vi "Camera.vi"(11 "test mode":bool) -> (1 "Error":bool)   [LabVIEW 2020]
panel:
  out "standard output":string caption="Standardausgabe"
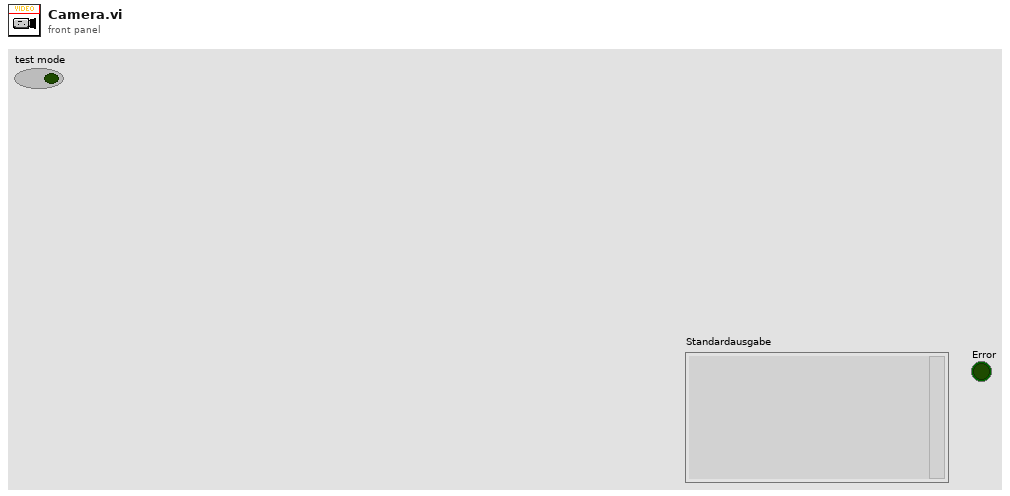
[diagram p1: front panel]
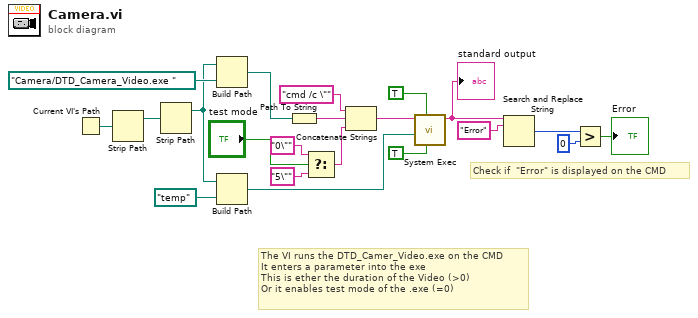
[diagram p0: block diagram]
diagram:
  # "Check if  \"Error\" is displayed on the CMD"
  # "The VI runs the DTD_Camer_Video.exe on the CMD\nIt enters a parameter into the exe\nThis is ether the duration of the Video (>0)\nOr it enables test mode of the .exe (=0)"
  n1 = Current VI's Path() -> (path=w10:path)
  n2 = Strip Path(path=w10) -> (stripped path=w9:path)  [unwired: 1 out]
  n3 = Strip Path(path=w9) -> (stripped path=w3:path)  [unwired: 1 out]
  n4 = Build Path(base path=w3, name or relative path=path "Camera/DTD_Camera_Video.exe ") -> (appended path=w18:path)
  n5 = Build Path(base path=w3, name or relative path=path "temp") -> (appended path=w1:path)
  n6 = Path To String(path=w18) -> (string=w17:string)
  n7 = Select(t="0\"" ("string"), s="test mode", f="5\"" ("string")) -> (s? t:f=w16:string)
  n8 = Concatenate Strings("cmd /c \"" ("string"), w17, w16) -> (w11:string)
  n9 = call <vilib>:"System Exec.vi"("run minimized? (F)"=TRUE, "wait until completion? (T)"=TRUE, "working directory"=w1, "command line"=w11) -> ("standard output"=w4:string)  [unwired: 4 in, 3 out]
  "standard output" <- w4
  n10 = Search and Replace String(input string=w4, search string="Error") -> (number of replacements=w7:i32)  [unwired: 6 in, 3 out]
  n11 = Greater?(x=w7, y=0) -> (0:→"Error":bool)
